vi "Add Event.vi"(8 "error in (no error)":errorcluster, 9 "Controller Event Fire Handler":refnum<class "Abstract Event Handler for Controller.lvclass">, 10 "Event":refnum<class "Event.lvclass">, 11 "Controller Actor in":refnum<class "Controller Actor.lvclass">) -> (0 "error out":errorcluster, 3 "Controller Actor out":refnum<class "Controller Actor.lvclass">)   [LabVIEW 2017, in "Event Actors.lvlib" / "Controller Actor.lvclass"]
doc: "This methods adds an event to the list of the events handled by the Controller. If the Controller wants to handle the events form the View, a \"Controller Event Fire Handler\" should be wired"
uses:
  Controller Actor.lvclass
  Event/Event.lvclass
  Event Handlers/Abstract Event Handler for Controller/Abstract Event Handler for Controller.lvclass
  Controller Actor.lvclass/Controller Actor.ctl
  <vilib>/Utility/error.llb/Error Cluster From Error Code.vi
  <vilib>/ErrorRing/Error Ring.xnode
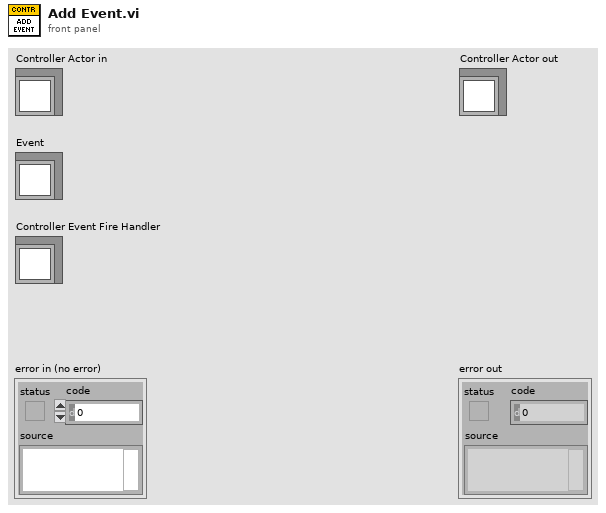
[diagram p1: front panel]
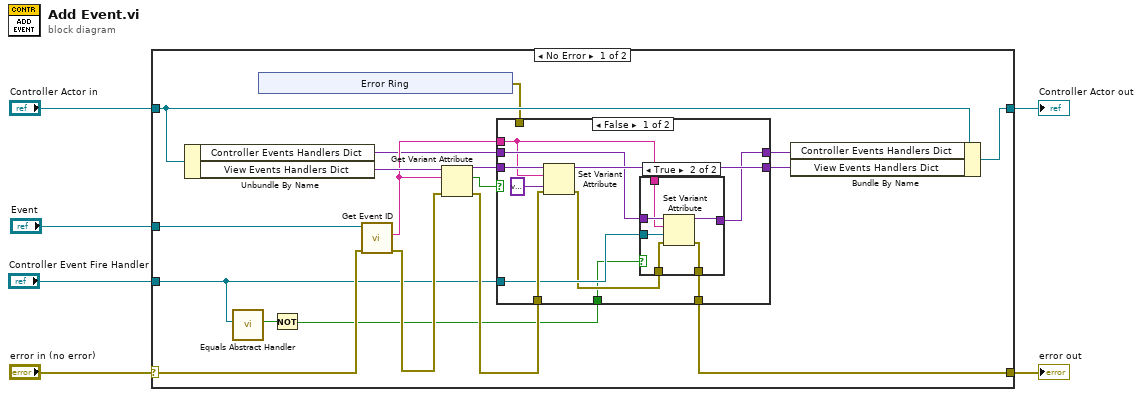
[diagram p0: block diagram]
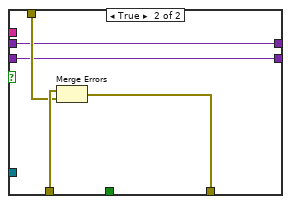
[diagram p3: hidden frame]
diagram:
  n1 = case shown="No Error" "error in (no error)" {
    selector: "error in (no error)" -> [w22 w54]
    tunnel: [w11 w54] -> w5
    tunnel: [w14 w53] -> w3
    tunnel: "Controller Actor in" -> [w24 w53]
    tunnel: "Event" -> [w23 _]
    tunnel: "Controller Event Fire Handler" -> [w9 _]
    frame No Error {
      n2 = Unbundle By Name(w24) -> ("Controller Events Handlers Dict"=w12:variant, "View Events Handlers Dict"=w21:variant)
      n3 = call "Equals Abstract Handler.vi"("Controller Event Fire Handler"=w9) -> ("Is Abstract Event Handler"=w8:bool)  [unwired: 10 in]
      n4 = xnode "Error Ring"() -> ("error out"=w15:errorcluster)
      n5 = Not(x=w8) -> (.not. x?=w7:bool)
      n6 = call-dynamic "Get Event ID.vi"("error in (no error)"=w22, "Event in"=w23) -> ("error out"=w20:errorcluster, "Event ID"=w17:string)  [unwired: 7 in, 1 out]
      n7 = Get Variant Attribute(Variant=w21, name=w17, error in=w20) -> (duplicate Variant=w18:variant, found=w19:bool, error out=w16:errorcluster)  [unwired: 1 in, 1 out]
      n8 = case shown="False" w19 {
        tunnel: w18 -> [w39 w50]
        tunnel: w17 -> [w34 _]
        tunnel: w16 -> [w38 w52]
        tunnel: w15 -> [_ w51]
        tunnel: [w36 w50] -> w13
        tunnel: w12 -> [w35 w48]
        tunnel: w9 -> [w33 _]
        tunnel: [w31 w49] -> w11
        tunnel: w7 -> [w30 _]
        tunnel: [w29 w48] -> w10
        frame False {
          n9 = Set Variant Attribute(Variant=w39, name=w34, value=variant ("Events Dict"), error in=w38) -> (Variant out=w36:variant, error out=w32:errorcluster)  [unwired: 1 out]
          n10 = case shown="True" w30 {
            tunnel: w35 -> [w40 w47]
            tunnel: w34 -> [_ w46]
            tunnel: w33 -> [_ w45]
            tunnel: w32 -> [w41 w44]
            tunnel: [w41 w43] -> w31
            tunnel: [w40 w42] -> w29
            frame False {
            }
            frame True {
              n11 = Set Variant Attribute(Variant=w47, name=w46, value=w45, error in=w44) -> (Variant out=w42:variant, error out=w43:errorcluster)  [unwired: 1 out]
            }
          }
        }
        frame True {
          n12 = Merge Errors(w52, w51) -> (w49:errorcluster)
        }
      }
      n13 = Bundle By Name(cluster=w24, "Controller Events Handlers Dict"=w10, "View Events Handlers Dict"=w13) -> (w14:refnum<class "Controller Actor.lvclass">)
    }
    frame Error {
    }
  }
  "error out" <- w5
  "Controller Actor out" <- w3
